vi "pxie_7962_fpga.vi"() -> ()   [LabVIEW 2014]
uses:
  <instrlib>/_niInstr/Streaming/v1/Common/Stream State.ctl
  <vilib>/Platform/TimedLoop/XDataNode/timing_clust.ctl
  <vilib>/Platform/TimedLoop/XDataNode/nitl_modes.ctl
  <vilib>/Platform/TimedLoop/XDataNode/wakeup.ctl
  FPGA_Controls/Acquisition FIFOs Cluster.ctl
  <vilib>/rvi/Emulation/niFpgaSctlEmulationGetInTimedLoop.vi
  <vilib>/rvi/Emulation/niFpgaEmulationReportErrorSimple.vi
  <vilib>/rvi/Emulation/niFpgaGetClockAttributes.vi
  <vilib>/rvi/Emulation/niFpgaCriticalErrorInLSC.vi
  <vilib>/rvi/eio/common/nirviEmuTemplateMethod_errors.vi
  <instrlib>/_niInstr/Basic Elements/v1/FPGA/Private/Count Up U32.vi
  <vilib>/rvi/Memory/Memory_Emulation/niFpgaMemoryFastEmulationDramWriteAndRequestData.vi
  <vilib>/rvi/Memory/Memory_Emulation/niFpgaMemoryEmulationDramWriteAndRequestData.vi
  <vilib>/rvi/DataTransferAndStorage/Container/Common/niFpgaContainerGetUniqueNameForEmu.vi
  <vilib>/rvi/Memory/Memory_Emulation/niFpgaMemoryEmulationDramWriteAndRequestDataApplyByteEnables.vi
  <vilib>/rvi/interface/RandomDataEmulation/niFpgaRandomDataHandleErrors.vi
  <instrlib>/_niInstr/Basic Elements/v1/FPGA/Private/Count Up U64.vi
  <vilib>/rvi/DataTransferAndStorage/Container/Common/niFpgaContainerExecOnDevCompGetState.vi
  <vilib>/rvi/Emulation/niFpgaEmulationIsFPGAContextNoSignature.vi
  <vilib>/rvi/errors/niFpgaSetErrorForExecOnDevCompSimple.vi
  <vilib>/rvi/eio/common/nirviEmuReportErrorAndStop.vi
  <vilib>/rvi/FIFO/Fifo_Resource/nirvififoEmulationSetSize.vi
  <vilib>/rvi/FIFO/Fifo_Resource/nirviFifoEmulationQueueMgr.vi
  <instcachedir>/0/nirviFifoEmulationQueueMgr_E5CAEC123FF24DC58D834DCA3CDAA9B5.lvgen/nirviFifoEmulationQueueMgr_E5CAEC123FF24DC58D834DCA3CDAA9B5_003.vi
  <vilib>/rvi/FIFO/Fifo_Resource/nirvififoEmulationDetermineInputValidOut.vi
  <vilib>/rvi/FIFO/Fifo_Resource/nirvififoEmulationCreateLock.vi
  <vilib>/rvi/Emulation/niFpgaProcessEmulError.vi
  <vilib>/rvi/FIFO/Fifo_Resource/nirvififoEmulationObtainLock.vi
  <vilib>/rvi/FIFO/Fifo_Resource/nirvififoEmulationReleaseLock.vi
  <vilib>/rvi/occurrence/nirviWaitOnOccurrenceBase.vi
  <vilib>/rvi/errors/nirviReportUnexpectedCaseInternalError.vi
  <vilib>/rvi/errors/nirviReportUnexpectedCaseInternalError (U32).vi
  <vilib>/Utility/error.llb/Clear Errors.vi
  <vilib>/Platform/TimedLoop/XDataNode/XDataNode.xnode
  <vilib>/eio/EIONode/EIONode.xnode
  <vilib>/rvi/DataTransferAndStorage/Container/XNode/niFpgaContainer.xnode
  <vilib>/rvi/Memory/Memory_Emulation/niFpgaMemoryEmulationDramRetrieveData.vi
  <vilib>/rvi/interface/RandomDataEmulation/nirviRandomDataFpgaReadWriteTemplate.vi
  <vilib>/rvi/FIFO/Fifo_Resource/niFpgaFifoEmulationRefIn.vi
  <vilib>/Platform/TimedLoop/XDataNode/XDNodeRunTimeDep.lvlib
  <instrlib>/_niInstr/Streaming/v1/FPGA/niInstr Streaming v1 FPGA.lvlib
  <instrlib>/_niInstr/Basic Elements/v1/FPGA/niInstr Basic Elements v1 FPGA.lvlib
  <instrlib>/_niInstr/Streaming/v1/Common/niInstr Streaming v1 Common.lvlib
panel:
  in  "manual\ntrigger":bool
  out "Writes to DRAM":u64
  out "DRAM Write address":u32
  in  "Reset DRAM write address":bool
  in  "Reset DRAM read address":bool
  in  "trigger \ndelay":u64
  in  "Clear Trigger":bool
  in  "Output Debug Data":bool
  out "stream.metadata 0":u64
  in  "stream.request state 0":T1
  out "stream.samples transferred 0":u64
  out "stream.state 0":T1
  in  "stream.num samples 0":u64
  out "Writes to DMA":u64
  out "Samples Aquired":u64
  out "IO Module Init Done":bool
  in  "stream.num samples 1":u64
  out "stream.state 1":T1
  out "stream.samples transferred 1":u64
  in  "stream.request state 1":T1
  out "stream.metadata 1":u64
  # "Stream 0 (Aquisition Stream)"
  # "Throughput Diagnostics"
  # "Stream 1 (Transfer to Host Stream)"
  # "Settings & Resets"
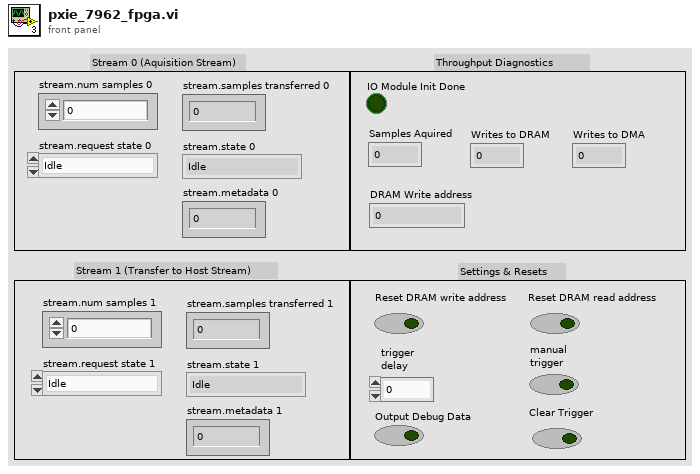
[diagram p1: front panel]
types:
  T1 = typedef "niInstr Streaming v1 Common.lvlib/Stream State.ctl" = enum8{"Idle", "Finite Transfer", "Continuous", "Done", "Error", "Not Ready", "Cancel"}
  T2 = typedef "XDNodeRunTimeDep.lvlib/timing_clust.ctl" = cluster{"Expected End [f-1]":u64, "Actual End [f-1]":u64, "Finished Late? [f-1]":bool, "Expected End [i-1]":u64, "Actual End [i-1]":u64, "Finished Late? [i-1]":bool, "Expected Start [i]":u64, "Actual Start [i]":u64, "Expected Start [f]":u64, "Actual Start [f]":u64, "Source Name":string, "Structure Name":string, "Period":i64, "Deadline":i64, "Offset":i64, "Start":i64, "Priority":i32, "Timeout":i32, "Mode":T3, "Wakeup Reason":T4, "Error":errorcluster, "Source Type":string, "Secondary Source Type":string, "Global End Time":u64, "Global Start Time":u64, "Frame Duration":u64, "Iteration Duration":u64, "Assigned CPU":i32, "I/O Scan Engine Mode":u32}
  T3 = typedef "XDNodeRunTimeDep.lvlib/nitl_modes.ctl" = enum32{"No Change", "Process missed periods, maintain original phase", "Discard missed periods, maintain original phase", "Process missed periods, ignore original phase", "Discard missed periods, ignore original phase"}
  T4 = typedef "XDNodeRunTimeDep.lvlib/wakeup.ctl" = enum32{"Normal", "Aborted", "Asynchronous wakeup", "Timing source error", "Timed loop error", "Timeout"}
  T5 = typedef "Acquisition FIFOs Cluster.ctl" = cluster{"FIFO 0":refnum<k21>, "FIFO 1":refnum<k21>, "FIFO 2":refnum<k21>, "FIFO 3":refnum<k21>, "FIFO 4":refnum<k21>, "FIFO 5":refnum<k21>, "FIFO 6":refnum<k21>, "FIFO 7":refnum<k21>}
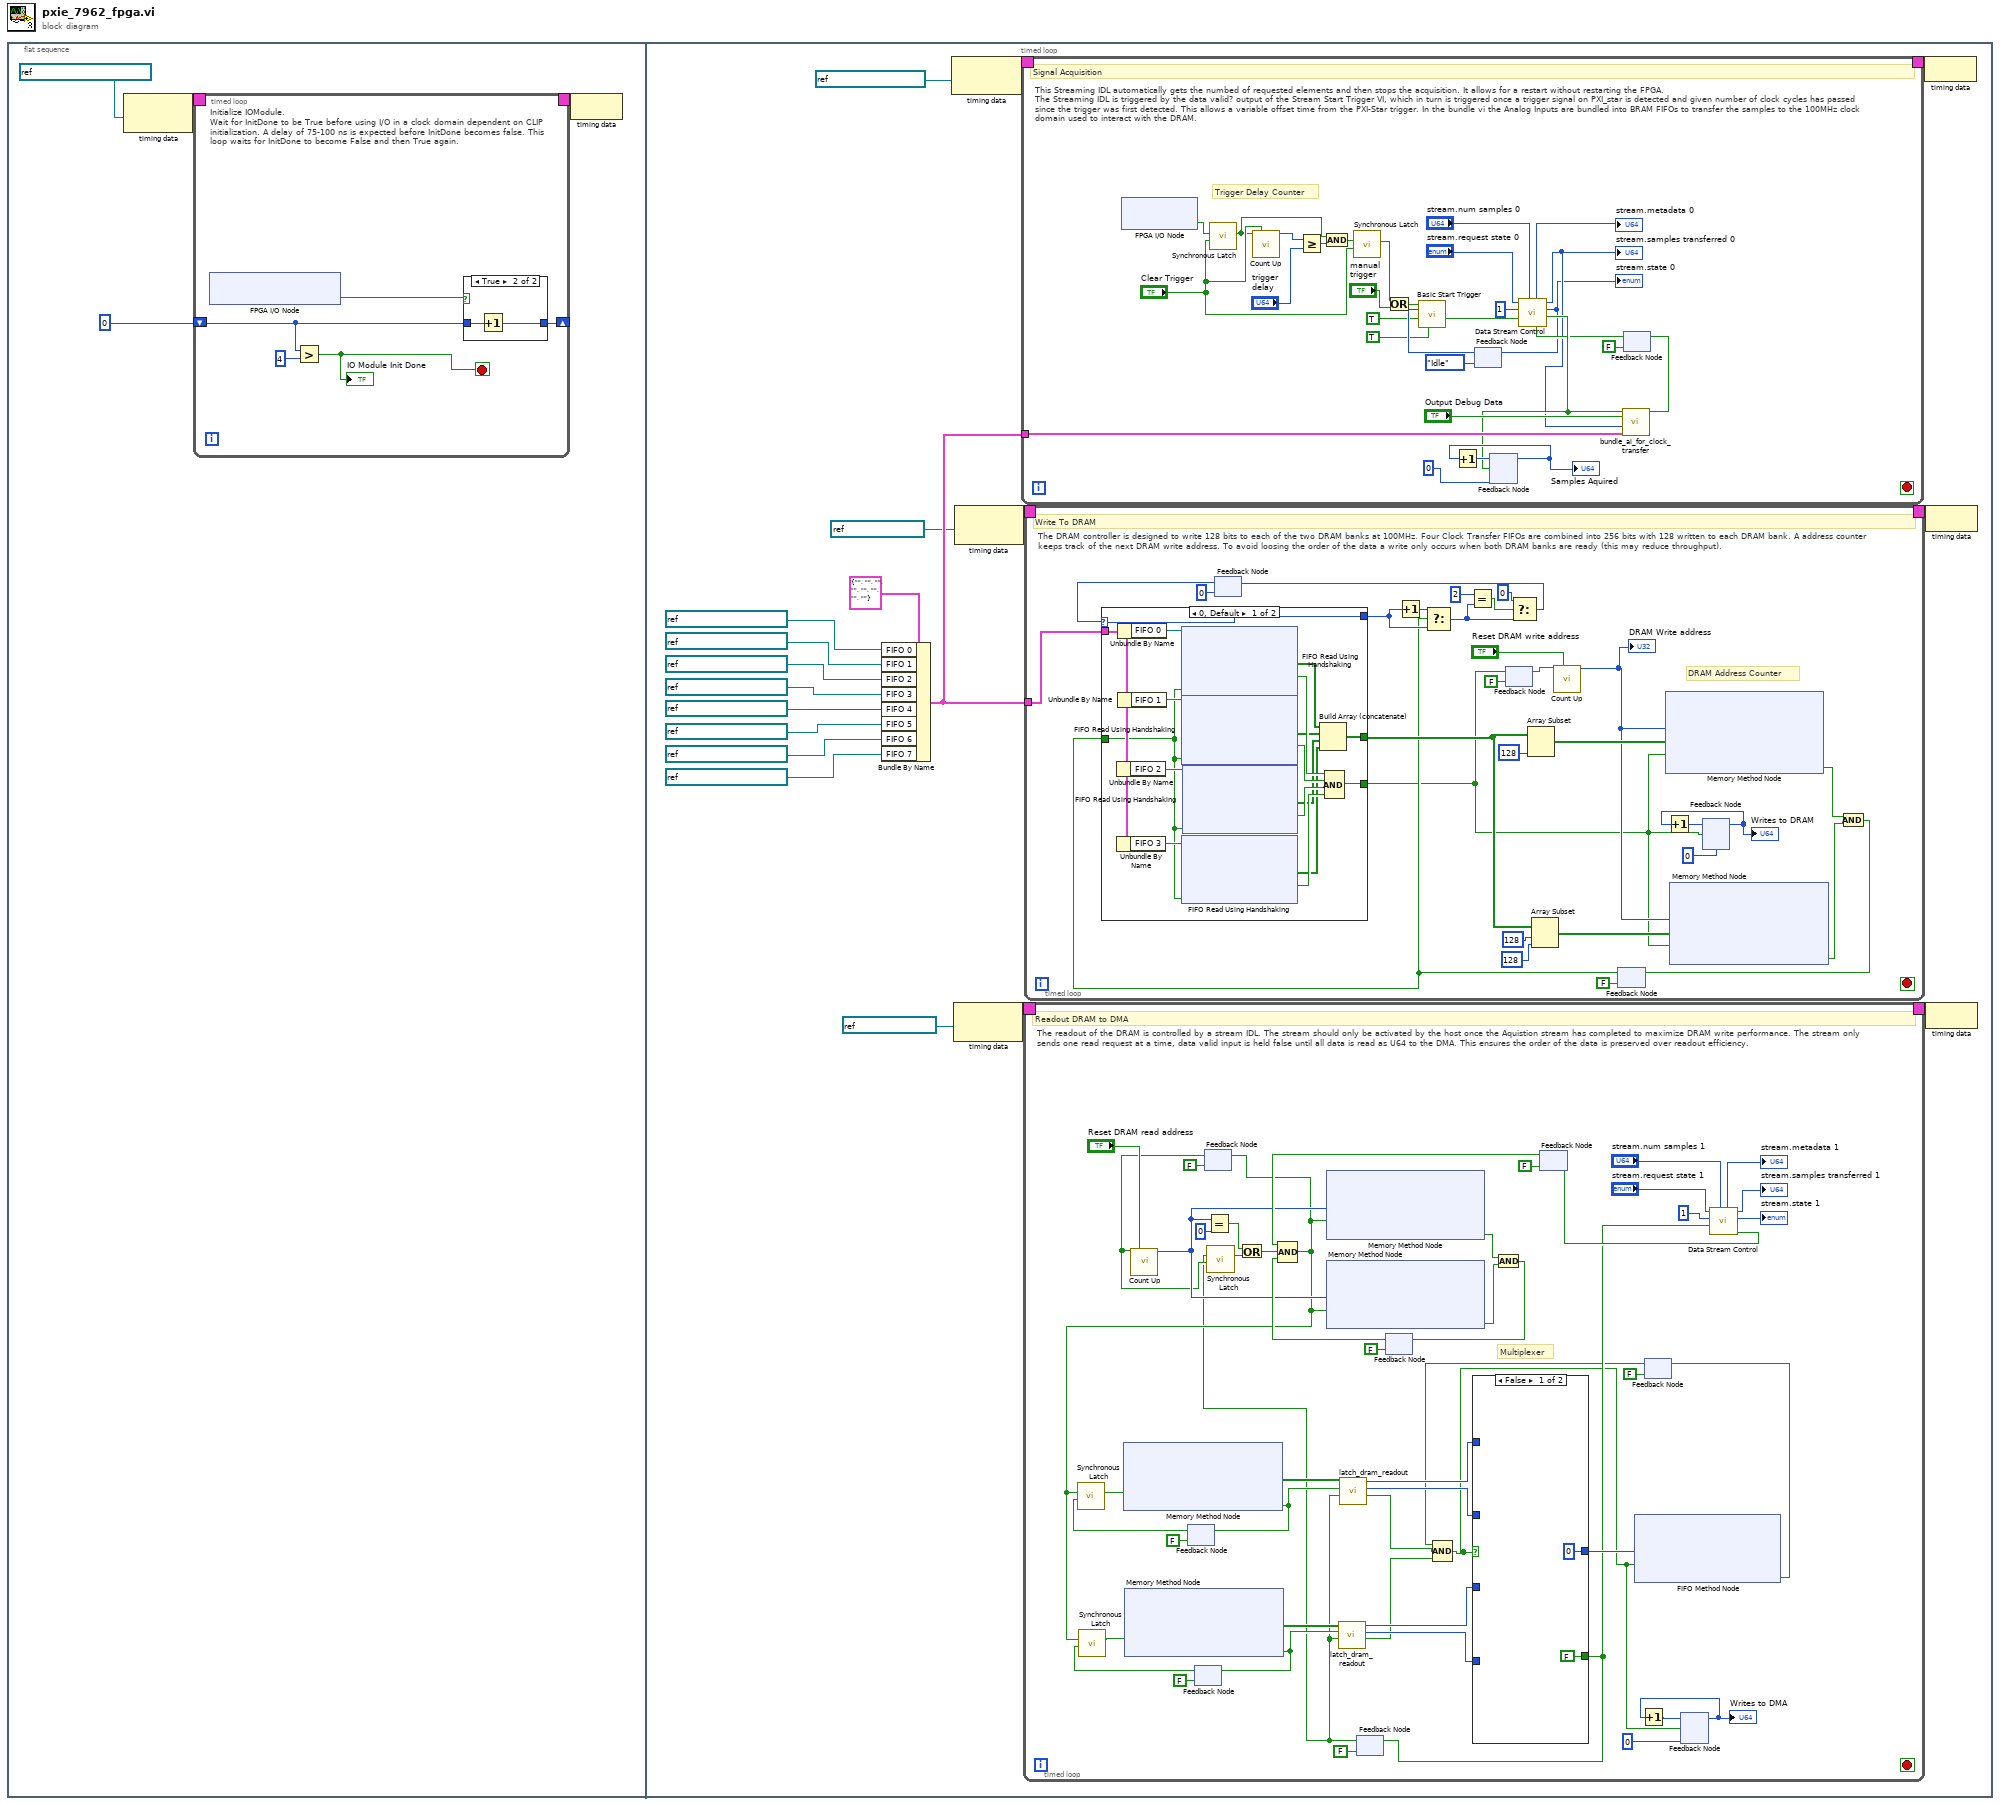
[diagram p0: block diagram]
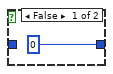
[diagram p2: hidden frame]
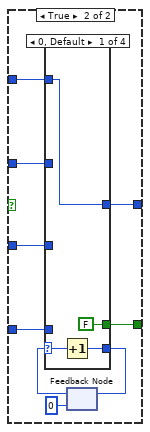
[diagram p3: hidden frame]
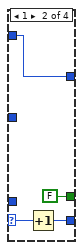
[diagram p4: hidden frame]
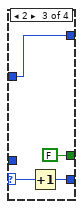
[diagram p5: hidden frame]
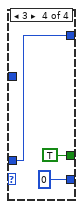
[diagram p6: hidden frame]
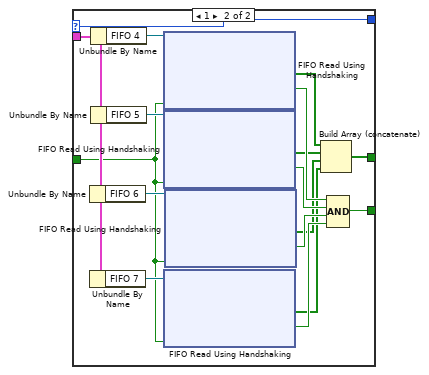
[diagram p7: hidden frame]
diagram:
  n1 = flat-sequence {
    frame #0 {
      n2 = node-c288(refnum<k21> "40 MHz Onboard Clock" ("Source Name")) -> (w4:T2)
      n3 = timed-loop {
        shift-right: [w9] -> _
        shift-left: u16 0 -> [w8]
        timing: w4 -> [_]
        timing-out: [_] -> w3
        stop <- w6 stop-if-true
        # "Initialize IOModule.\nWait for InitDone to be True before using I/O in a clock domain dependent on CLIP initialization. A delay of 75-100 ns is expected before InitDone becomes false. This loop waits for InitDone to become False and then True again."
        n4 = xnode "FPGA I/O Node"() -> ("IO Module\\InitDone"=w5:bool)  [unwired: 1 in, 1 out]
        n5 = Greater?(x=w8, y=u16 4) -> (0:w6:bool)
        "IO Module Init Done" <- w6
        n6 = case shown="True" w5 {
          tunnel: [u16 0 w12] -> w9
          tunnel: w8 -> [_ w11]
          frame False {
          }
          frame True {
            n7 = Increment(x=w11) -> (x+1=w12:u16)
          }
        }
      }
      n8 = node-c288(w3) -> ()
    }
    frame #1 {
      n9 = Bundle By Name(cluster=T5 {"FIFO 0"="", "FIFO 1"="", "FIFO 2"="", "FIFO 3"="", "FIFO 4"="", "FIFO 5"="", "FIFO 6"="", "FIFO 7"=""} ("FIFO Refs"), "FIFO 0"=refnum<k21> "Clock Transfer FIFO 0" ("FIFO In"), "FIFO 1"=refnum<k21> "Clock Transfer FIFO 1" ("FIFO In"), "FIFO 2"=refnum<k21> "Clock Transfer FIFO 2" ("FIFO In"), "FIFO 3"=refnum<k21> "Clock Transfer FIFO 3" ("FIFO In"), "FIFO 4"=refnum<k21> "Clock Transfer FIFO 4" ("FIFO In"), "FIFO 5"=refnum<k21> "Clock Transfer FIFO 5" ("FIFO In"), "FIFO 6"=refnum<k21> "Clock Transfer FIFO 6" ("FIFO In"), "FIFO 7"=refnum<k21> "Clock Transfer FIFO 7" ("FIFO In")) -> (w22:T5)
      n10 = node-c288(refnum<k21> "IO Module Clock 0" ("Source Name")) -> (w37:T2)
      n11 = node-c288(refnum<k21> "100 MHz Clock" ("Source Name")) -> (w33:T2)
      n12 = node-c288(refnum<k21> "100 MHz Clock" ("Source Name")) -> (w35:T2)
      n13 = timed-loop {
        timing: w37 -> [_]
        timing-out: [_] -> w36
        tunnel: w22 -> [w213]
        stop <- _ stop-if-true
        # "Trigger Delay Counter"
        # "This Streaming IDL automatically gets the numbed of requested elements and then stops the acquisition. It allows for a restart without restarting the FPGA. \nThe Streaming IDL is triggered by the data valid? output of the Stream Start Trigger VI, which in turn is triggered once a trigger signal on PXI_star is detected and given number of clock cycles has passed since the trigger was first detected. This allows a variable offset time from the PXI-Star trigger. In the bundle vi the Analog Inputs are bundled into BRAM FIFOs to transfer the samples to the 100MHz clock domain used to interact with the DRAM."
        # "Signal Acquisition"
        n14 = xnode "FPGA I/O Node"() -> ("PXI_Star"=w199:bool)  [unwired: 1 in, 1 out]
        n15 = call <instrlib>:"Synchronous Latch.vi"("clear"="Clear Trigger", "set"=w199) -> ("out"=w193:bool)  [unwired: 9 in]
        n16 = call-poly <instrlib>:"Count Up.vi"("increment"=w193, "reset"="Clear Trigger") -> ("count out"=w198:u64)  [unwired: 13 in]
        n17 = Greater Or Equal?(x=w198, y="trigger \ndelay") -> (x >= y?=w194:bool)
        n18 = And(x=w193, y=w194) -> (x .and. y?=w192:bool)
        n19 = call <instrlib>:"Synchronous Latch.vi"("clear"="Clear Trigger", "set"=w192) -> ("out"=w191:bool)  [unwired: 9 in]
        n20 = Or(x=w191, y="manual\ntrigger") -> (x .or. y?=w189:bool)
        n21 = feedback #1(Stream_State."Idle" ("stream.state 0")) -> (w203:T1)
        n22 = call <instrlib>:"Basic Start Trigger.vi"("ready for start trigger"=TRUE, "data valid?"=TRUE, "stream.state"=w203, "start trigger"=w189) -> ("data valid"=w196:bool)  [unwired: 7 in]
        n23 = feedback #2(u64 0) -> (w214:u64)
        "Samples Aquired" <- w214
        n24 = Increment(x=w214) -> (x+1=w215:u64)
        n25 = feedback #3(FALSE ("Ready for Input")) -> (w210:bool)
        n26 = call <instrlib>:"Data Stream Control.vi"("ready for input?"=w210, "stream.num samples 0"="stream.num samples 0", "data valid"=w196, "element count"=u16 1, "stream.request state 0"="stream.request state 0") -> ("send data"=w211:bool, "stream.state 0"=w207:T1, "stream.samples transferred 0"=w208:u64, "stream.metadata 0"=→"stream.metadata 0":u64)  [unwired: 2 in, 1 out]
        "stream.state 0" <- w207
        "stream.samples transferred 0" <- w208
        n27 = feedback-in #1(w207) -> ()
        n28 = feedback-in #2(w215, w211) -> ()
        n29 = call "bundle_ai_for_clock_transfer.vi"("FIFO Refs"=w213, "sample"=w208, "Debug"="Output Debug Data", "Input Valid"=w211) -> ("Ready for Input"=w218:bool)  [unwired: 7 in]
        n30 = feedback-in #3(w218) -> ()
      }
      n31 = timed-loop {
        timing: w33 -> [_]
        timing-out: [_] -> w32
        stop <- _ stop-if-true
        # "Multiplexer"
        # "The readout of the DRAM is controlled by a stream IDL. The stream should only be activated by the host once the Aquistion stream has completed to maximize DRAM write performance. The stream only sends one read request at a time, data valid input is held false until all data is read as U64 to the DMA. This ensures the order of the data is preserved over readout efficiency."
        # "Readout DRAM to DMA"
        n32 = feedback #4(FALSE ("Output Valid")) -> (w52:bool)
        n33 = feedback #5(FALSE ("Output Valid")) -> (w49:bool)
        n34 = feedback #6(FALSE) -> (w59:bool)
        n35 = call-poly <instrlib>:"Count Up.vi"("increment"=w59, "reset"="Reset DRAM read address") -> ("count out"=w64:u32)  [unwired: 13 in]
        n36 = Equal?(x=w64, y=u32 0) -> (x = y?=w61:bool)
        n37 = feedback #7(FALSE) -> (w45:bool)
        n38 = call <instrlib>:"Synchronous Latch.vi"("clear"=w59, "set"=w45) -> ("out"=w60:bool)  [unwired: 9 in]
        n39 = Or(x=w61, y=w60) -> (x .or. y?=w62:bool)
        n40 = feedback #8(FALSE) -> (w66:bool)
        n41 = feedback #9(FALSE ("request data")) -> (w65:bool)
        n42 = Compound Arithmetic op=AND(w65, w62, w66) -> (w48:bool)
        n43 = call <instrlib>:"Synchronous Latch.vi"("clear"=w52, "set"=w48) -> ("out"=w55:bool)  [unwired: 9 in]
        n44 = call <instrlib>:"Synchronous Latch.vi"("clear"=w49, "set"=w48) -> ("out"=w54:bool)  [unwired: 9 in]
        n45 = xnode ("Memory Method Node")("Ready for Output"=w55) -> ("Data"=w78:bool[], "Output Valid"=w53:bool)  [unwired: 1 in, 1 out]
        n46 = xnode ("Memory Method Node")("Ready for Output"=w54) -> ("Data"=w47:bool[], "Output Valid"=w46:bool)  [unwired: 1 in, 1 out]
        n47 = feedback-in #4(w53) -> ()
        n48 = feedback-in #5(w46) -> ()
        n49 = feedback-in #6(w48) -> ()
        n50 = xnode ("Memory Method Node")("Address"=w64, "Input Valid"=w48) -> ("Ready for Input"=w70:bool)  [unwired: 1 in, 1 out]
        n51 = xnode ("Memory Method Node")("Address"=w64, "Input Valid"=w48) -> ("Ready for Input"=w69:bool)  [unwired: 1 in, 1 out]
        n52 = call "latch_dram_readout.vi"("Reset"=w45, "Output Valid"=w46, "Data"=w47) -> ("Lateched Output Valid"=w38:bool, "latched U64 1"=w43:u64, "lateched U64 0"=w44:u64)  [unwired: 6 in]
        n53 = call "latch_dram_readout.vi"("Reset"=w45, "Output Valid"=w53, "Data"=w78) -> ("Lateched Output Valid"=w39:bool, "latched U64 1"=w77:u64, "lateched U64 0"=w76:u64)  [unwired: 6 in]
        n54 = And(x=w70, y=w69) -> (x .and. y?=w68:bool)
        n55 = feedback-in #8(w68) -> ()
        n56 = feedback #10(FALSE ("Ready for Input")) -> (w40:bool)
        n57 = Compound Arithmetic op=AND(w40, w39, w38) -> (w41:bool)
        n58 = case shown="False" w41 {
          tunnel: w43 -> [_ w98]
          tunnel: w44 -> [_ w97]
          tunnel: w77 -> [_ w96]
          tunnel: w76 -> [_ w95]
          tunnel: [u64 0 ("q") w91] -> w74
          tunnel: [FALSE w90] -> w58
          frame False {
          }
          frame True {
            n59 = feedback #11(i16 0) -> (w92:i16)
            n60 = case shown="0, Default" w92 {
              selector: w92 -> [w101 w105 w109 _]
              tunnel: w98 -> [_ _ _ w112]
              tunnel: w97 -> [_ _ w108 _]
              tunnel: w96 -> [_ w104 _ _]
              tunnel: w95 -> [w100 _ _ _]
              tunnel: [w102 w106 w110 i16 0] -> w94
              tunnel: [w100 w104 w108 w112] -> w91
              tunnel: [FALSE FALSE FALSE TRUE] -> w90
              frame 0, Default {
                n61 = Increment(x=w101) -> (x+1=w102:i16)
              }
              frame 1 {
                n62 = Increment(x=w105) -> (x+1=w106:i16)
              }
              frame 2 {
                n63 = Increment(x=w109) -> (x+1=w110:i16)
              }
              frame 3 {
              }
            }
            n64 = feedback-in #11(w94) -> ()
          }
        }
        n65 = feedback-in #7(w58) -> ()
        n66 = xnode ("FIFO Method Node")("Element"=w74, "Input Valid"=w41) -> ("Ready for Input"=w75:bool)  [unwired: 1 in, 1 out]
        n67 = feedback-in #10(w75) -> ()
        n68 = feedback #12(u64 0) -> (w81:u64)
        "Writes to DMA" <- w81
        n69 = Increment(x=w81) -> (x+1=w82:u64)
        n70 = feedback-in #12(w82, w41) -> ()
        n71 = call <instrlib>:"Data Stream Control.vi"("stream.num samples 0"="stream.num samples 1", "data valid"=w58, "element count"=u16 1, "stream.request state 0"="stream.request state 1") -> ("request data"=w72:bool, "stream.state 0"=→"stream.state 1":T1, "stream.samples transferred 0"=→"stream.samples transferred 1":u64, "stream.metadata 0"=→"stream.metadata 1":u64)  [unwired: 3 in, 1 out]
        n72 = feedback-in #9(w72) -> ()
      }
      n73 = timed-loop {
        timing: w35 -> [_]
        timing-out: [_] -> w34
        tunnel: w22 -> [w148]
        stop <- _ stop-if-true
        # "DRAM Address Counter"
        # "The DRAM controller is designed to write 128 bits to each of the two DRAM banks at 100MHz. Four Clock Transfer FIFOs are combined into 256 bits with 128 written to each DRAM bank. A address counter keeps track of the next DRAM write address. To avoid loosing the order of the data a write only occurs when both DRAM banks are ready (this may reduce throughput)."
        # "Write To DRAM"
        n74 = feedback #13(i16 0 ("t")) -> (w147:i16)
        n75 = feedback #14(FALSE ("Output Valid")) -> (w128:bool)
        n76 = call-poly <instrlib>:"Count Up.vi"("increment"=w128, "reset"="Reset DRAM write address") -> ("count out"=w127:u32)  [unwired: 13 in]
        "DRAM Write address" <- w127
        n77 = feedback #15(FALSE) -> (w124:bool)
        n78 = case shown="0, Default" w147 {
          selector: w147 -> [w164 w181]
          tunnel: w148 -> [w150 w167]
          tunnel: [w162 w179] -> w125
          tunnel: [w155 w172] -> w120
          tunnel: [w164 w181] -> w145
          tunnel: w124 -> [w149 w166]
          frame 0, Default {
            n79 = Unbundle By Name(w150) -> ("FIFO 2"=w161:refnum<k21>)
            n80 = Unbundle By Name(w150) -> ("FIFO 3"=w160:refnum<k21>)
            n81 = Unbundle By Name(w150) -> ("FIFO 0"=w165:refnum<k21>)
            n82 = Unbundle By Name(w150) -> ("FIFO 1"=w163:refnum<k21>)
            n83 = xnode ("FIFO Read Using Handshaking")("Ready for Output"=w149, "FIFO In"=w165) -> ("Element"=w154:bool[], "Output Valid"=w159:bool)  [unwired: 1 out]
            n84 = xnode ("FIFO Read Using Handshaking")("Ready for Output"=w149, "FIFO In"=w163) -> ("Element"=w153:bool[], "Output Valid"=w158:bool)  [unwired: 1 out]
            n85 = xnode ("FIFO Read Using Handshaking")("Ready for Output"=w149, "FIFO In"=w160) -> ("Element"=w151:bool[], "Output Valid"=w156:bool)  [unwired: 1 out]
            n86 = xnode ("FIFO Read Using Handshaking")("Ready for Output"=w149, "FIFO In"=w161) -> ("Element"=w152:bool[], "Output Valid"=w157:bool)  [unwired: 1 out]
            n87 = Build Array (concatenate)(w154, w153, w152, w151) -> (w162:bool[])
            n88 = Compound Arithmetic op=AND(w159, w158, w157, w156) -> (w155:bool)
          }
          frame 1 {
            n89 = Unbundle By Name(w167) -> ("FIFO 6"=w178:refnum<k21>)
            n90 = Unbundle By Name(w167) -> ("FIFO 7"=w177:refnum<k21>)
            n91 = Unbundle By Name(w167) -> ("FIFO 4"=w182:refnum<k21>)
            n92 = Unbundle By Name(w167) -> ("FIFO 5"=w180:refnum<k21>)
            n93 = xnode ("FIFO Read Using Handshaking")("Ready for Output"=w166, "FIFO In"=w182) -> ("Element"=w171:bool[], "Output Valid"=w176:bool)  [unwired: 1 out]
            n94 = xnode ("FIFO Read Using Handshaking")("Ready for Output"=w166, "FIFO In"=w180) -> ("Element"=w170:bool[], "Output Valid"=w175:bool)  [unwired: 1 out]
            n95 = xnode ("FIFO Read Using Handshaking")("Ready for Output"=w166, "FIFO In"=w177) -> ("Element"=w168:bool[], "Output Valid"=w173:bool)  [unwired: 1 out]
            n96 = xnode ("FIFO Read Using Handshaking")("Ready for Output"=w166, "FIFO In"=w178) -> ("Element"=w169:bool[], "Output Valid"=w174:bool)  [unwired: 1 out]
            n97 = Build Array (concatenate)(w171, w170, w169, w168) -> (w179:bool[])
            n98 = Compound Arithmetic op=AND(w176, w175, w174, w173) -> (w172:bool)
          }
        }
        n99 = Increment(x=w145) -> (x+1=w146:i16)
        n100 = Select(t=w146, s=w124, f=w145) -> (s? t:f=w143:i16)
        n101 = Equal?(x=i16 2, y=w143) -> (x = y?=w142:bool)
        n102 = feedback-in #14(w120) -> ()
        n103 = Select(t=i16 0, s=w142, f=w143) -> (s? t:f=w141:i16)
        n104 = feedback-in #13(w141) -> ()
        n105 = Array Subset(array=w125, length=128) -> (w134:bool[])  [unwired: 1 in]
        n106 = Array Subset(array=w125, index=128, length=128) -> (w133:bool[])
        n107 = xnode ("Memory Method Node")("Address"=w127, "Data"=w134, "Input Valid"=w120) -> ("Ready for Input"=w131:bool)  [unwired: 1 in, 1 out]
        n108 = xnode ("Memory Method Node")("Address"=w127, "Data"=w133, "Input Valid"=w120) -> ("Ready for Input"=w132:bool)  [unwired: 1 in, 1 out]
        n109 = feedback #16(u64 0) -> (w122:u64)
        "Writes to DRAM" <- w122
        n110 = Increment(x=w122) -> (x+1=w123:u64)
        n111 = feedback-in #16(w123, w120) -> ()
        n112 = And(x=w131, y=w132) -> (x .and. y?=w130:bool)
        n113 = feedback-in #15(w130) -> ()
      }
      n114 = node-c288(w36) -> ()
      n115 = node-c288(w34) -> ()
      n116 = node-c288(w32) -> ()
    }
  }
